vi "userEditAmount.vi"(8 "error in (no error)":errorcluster, 11 "Category In":refnum<class "Category.lvclass">) -> (0 "error out":errorcluster, 2 "UserConfirm?":bool, 3 "Category Out":refnum<class "Category.lvclass">)   [LabVIEW 2018, in "Category.lvclass"]
uses:
  Category.lvclass
  Category.lvclass/Category.ctl
panel:
  in  "Ok":bool
  in  "Amount":dbl
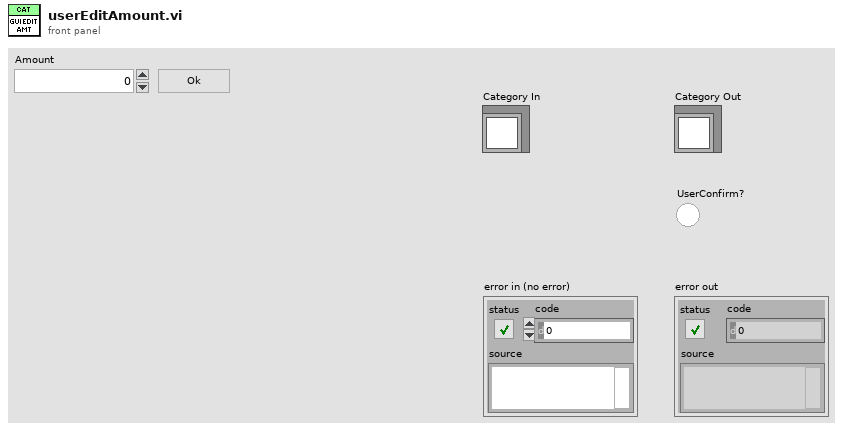
[diagram p1: front panel]
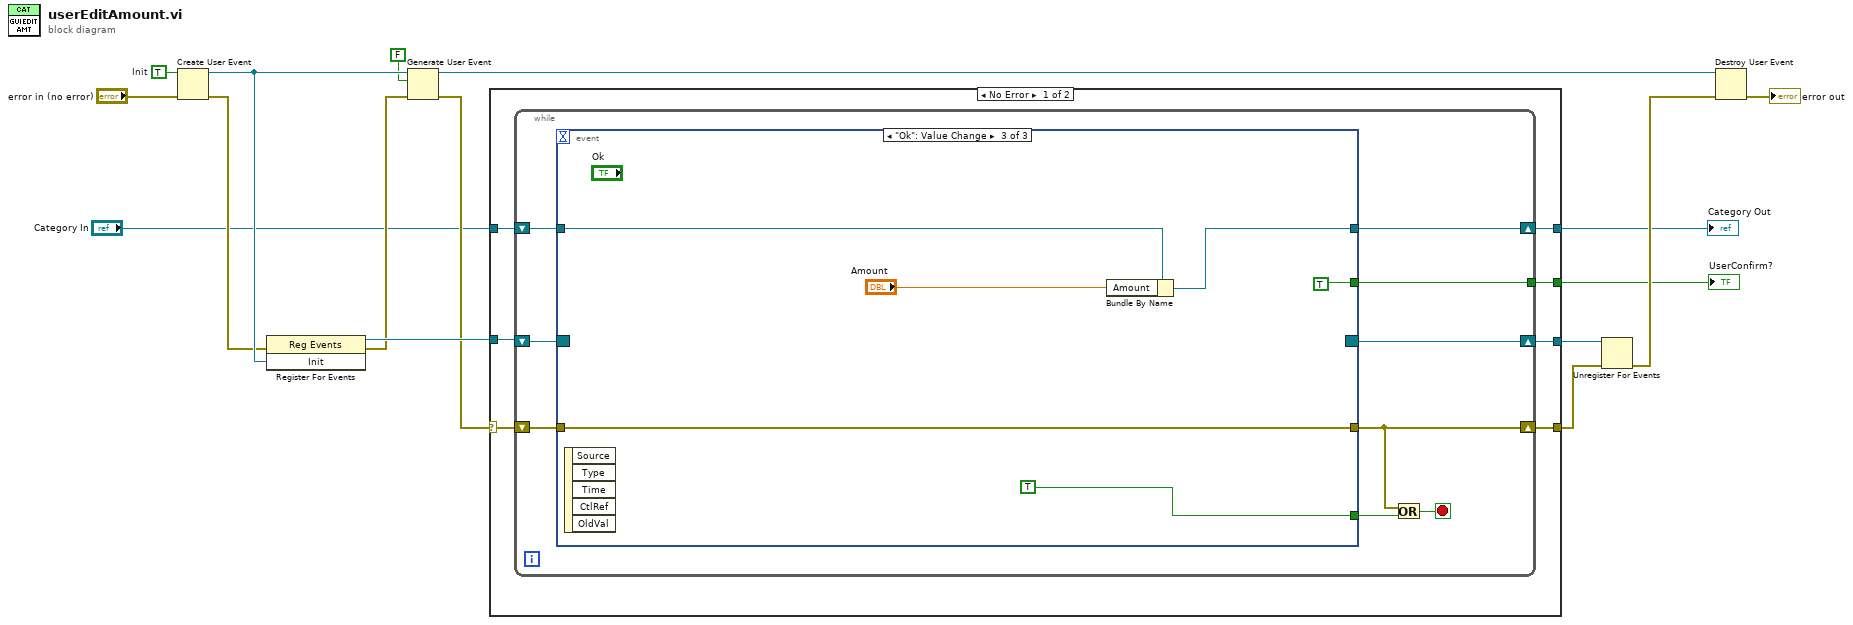
[diagram p0: block diagram]
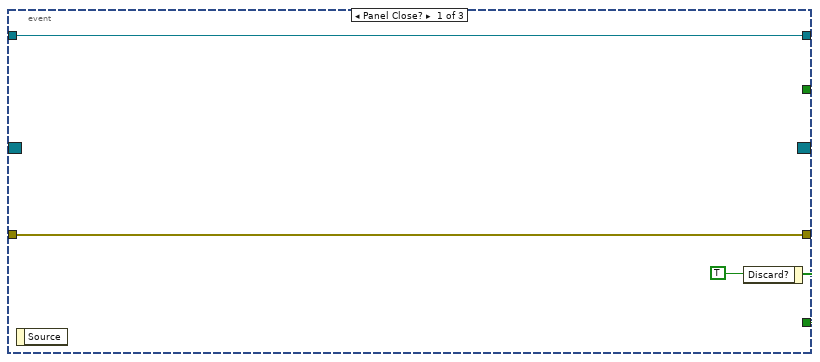
[diagram p2: hidden frame]
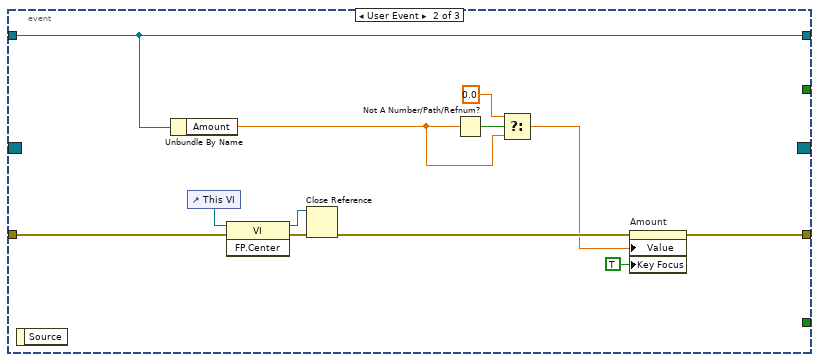
[diagram p3: hidden frame]
diagram:
  w16 = TRUE  # Init
  n1 = Create User Event(user event datatype=w16, error in="error in (no error)") -> (user event=w14:refnum<user-event>, error out=w11:errorcluster)
  n2 = register-events(error in=w11, w14) -> (reference out=w15:refnum<event-registration>, error out=w13:errorcluster)  [unwired: 1 in]
  n3 = Generate User Event(user event=w14, event data cluster=FALSE ("event data"), error in=w13) -> (user event out=w10:refnum<user-event>, error out=w3:errorcluster)  [unwired: 1 in]
  n4 = case shown="No Error" w3 {
    selector: w3 -> [w17 w56]
    tunnel: w15 -> [w23 w55]
    tunnel: [w22 w55] -> w9
    tunnel: [w21 w56] -> w8
    tunnel: [w20 w54] -> w1
    tunnel: "Category In" -> [w19 w54]
    tunnel: [w18 _] -> w4
    frame No Error {
      n5 = while {
        shift-right: [w30] -> w22
        shift-left: w23 -> [w32]
        shift-right: [w29] -> w21
        shift-left: w17 -> [w31]
        tunnel: [w24] -> w18
        shift-right: [w26] -> w20
        shift-left: w19 -> [w25]
        stop <- w27 stop-if-true
        n6 = event shown="[2] \"Ok\": Value Change" {
          selector: w32 -> [_ _ _]
          dyn-events: [_ _ _] -> w30
          timeout: _ -> [_ _ _]
          tunnel: [w35 _ TRUE ("Discard?")] -> w28
          tunnel: w31 -> [w34 w46 w52]
          tunnel: [w34 w43 w52] -> w29
          tunnel: [w33 w37 w49] -> w26
          tunnel: w25 -> [w33 w37 w50]
          tunnel: [_ _ TRUE ("Discard?")] -> w24
          event Panel Close? {
            w35 = TRUE ("Discard?")
            n7 = event-data() -> ()  [unwired: 1 in, 1 out]
            n8 = event-data("Discard?"=w35) -> ()  [unwired: 1 in, 1 out]
          }
          event User Event {
            n9 = event-data() -> ()  [unwired: 1 in, 1 out]
            n10 = Unbundle By Name(w37) -> ("Amount"=w36:dbl)
            n11 = control-ref of="This VI"() -> (w47:refnum<vi>)
            n12 = invoke class="VI" method="FP.Center"(reference=w47, error in=w46) -> (reference out=w44:refnum<vi>, error out=w45:errorcluster)  [unwired: 1 in, 1 out]
            n13 = Close Reference(reference=w44, error in (no error)=w45) -> (error out=w41:errorcluster)
            n14 = Not A Number/Path/Refnum?(number/path/refnum=w36) -> (NaN/Path/Refnum?=w40:bool)
            n15 = Select(t=0.0, s=w40, f=w36) -> (s? t:f=w39:dbl)
            n16 = property on="Amount" class="DigNum (strict)"(error in=w41, "Value"=w39, "Key Focus"=TRUE) -> (error out=w43:errorcluster)  [unwired: 1 in, 1 out]
          }
          event "Ok": Value Change {
            n17 = event-data() -> ()  [unwired: 1 in, 5 out]
            n18 = Bundle By Name(cluster=w50, "Amount"="Amount") -> (w49:refnum<class "Category.lvclass">)
          }
        }
        n19 = Or(x=w29, y=w28) -> (x .or. y?=w27:bool)
      }
    }
    frame Error {
    }
  }
  "UserConfirm?" <- w4
  "Category Out" <- w1
  n20 = Unregister For Events(event registration refnum=w9, error in=w8) -> (error out=w6:errorcluster)
  n21 = Destroy User Event(user event=w10, error in=w6) -> (error out=→"error out":errorcluster)
